vi "delete Init RefreshTime Notifier.vi"(8 "error in (no error)":errorcluster, 11 "Transport in":refnum<class "Transport.lvclass">) -> (0 "error out":errorcluster, 3 "Transport out":refnum<class "Transport.lvclass">)   [LabVIEW 2019]
uses:
  Transport.lvclass
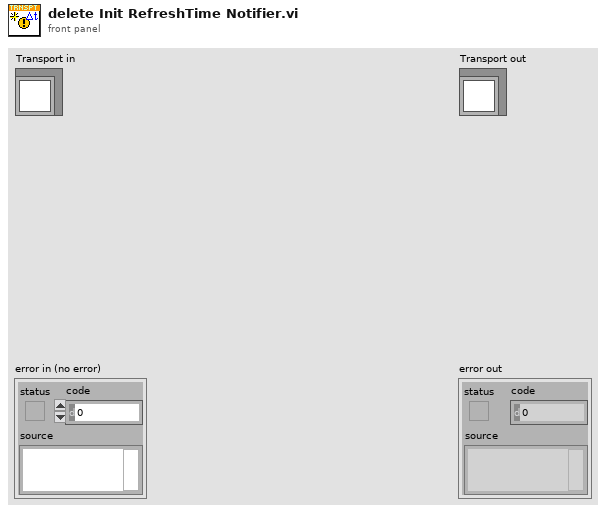
[diagram p1: front panel]
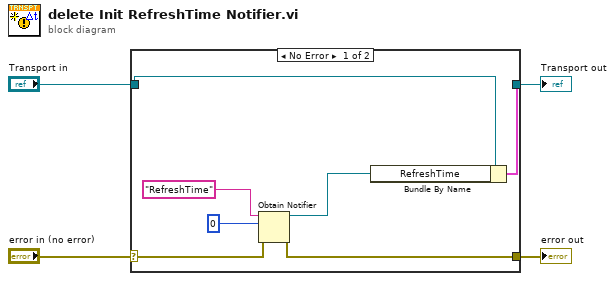
[diagram p0: block diagram]
diagram:
  n1 = case shown="No Error" "error in (no error)" {
    selector: "error in (no error)" -> [w6 w12]
    tunnel: [w5 w12] -> w3
    tunnel: [w10 w13] -> w1
    tunnel: "Transport in" -> [w11 w13]
    frame No Error {
      n2 = Obtain Notifier(name (unnamed)="RefreshTime", notification data type=u32 0, error in (no error)=w6) -> (notifier out=w8:refnum<notifier>, error out=w5:errorcluster)  [unwired: 1 in, 1 out]
      n3 = Bundle By Name(cluster=w11, "RefreshTime"=w8) -> (w10:cluster{})
    }
    frame Error {
    }
  }
  "error out" <- w3
  "Transport out" <- w1
